vi "전체_Selecter_Indexer.vi"(11 "전체_Selected":i32[](array[numeric])) -> (3 "Selected_Index":i32[](array[numeric]))   [LabVIEW 2014]
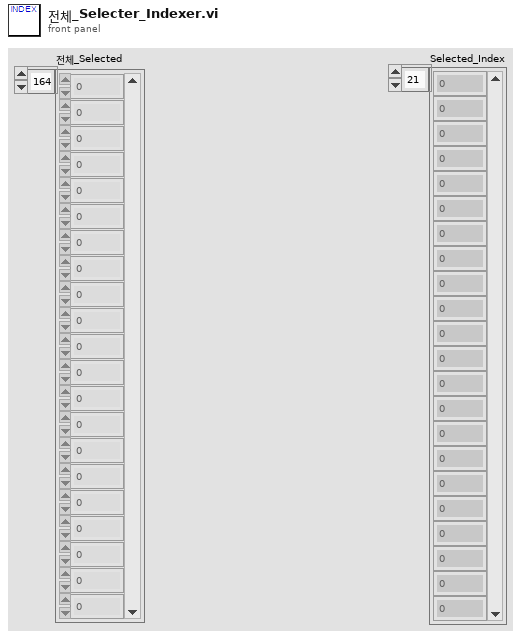
[diagram p1: front panel]
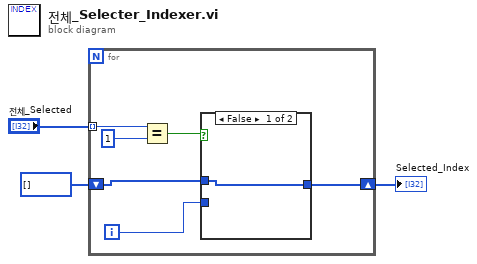
[diagram p0: block diagram]
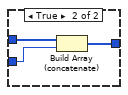
[diagram p2: hidden frame]
diagram:
  n1 = for {
    tunnel: "전체_Selected" -> [w9] mode=indexing
    shift-right: [w6] -> w1
    shift-left: i32[] [] -> [w5]
    i -> [w7]
    n2 = Equal?(x=w9, y=1) -> (x = y?=w8:bool)
    n3 = case shown="False" w8 {
      tunnel: w7 -> [_ w13]
      tunnel: [w10 w12] -> w6
      tunnel: w5 -> [w10 w11]
      frame False {
      }
      frame True {
        n4 = Build Array (concatenate)(w11, w13) -> (w12:i32[])
      }
    }
  }
  "Selected_Index" <- w1
